vi "TTA_MATLAB_Set_MATLAB_Path.vi"(8 "error in":errorcluster, 11 "MATLAB Directory":path=path "C:/Users/Alex.Minicozzi.NJ01/Documents/LabVIEW Data/BDS_MATLAB/ViennaGUI") -> (0 "error out":errorcluster)   [LabVIEW 2016]
uses:
  TTA_Globals/Test_Environment.vi
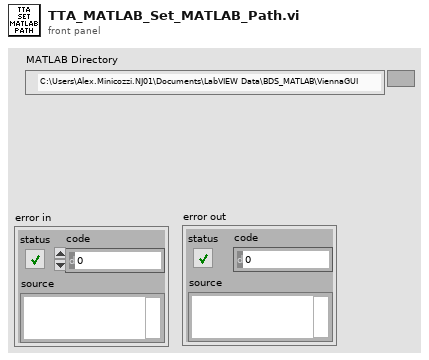
[diagram p1: front panel]
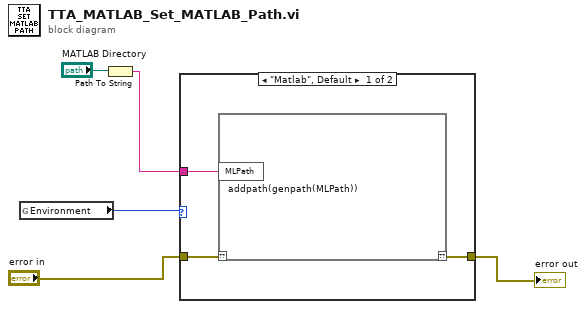
[diagram p0: block diagram]
diagram:
  n1 = global read "Test_Environment.vi" "Environment"() -> (w1:enum16{"Matlab", "LabVIEW"})
  n2 = Path To String(path="MATLAB Directory") -> (string=w2:string)
  n3 = case shown="\"Matlab\", Default" w1 {
    tunnel: "error in" -> [w8 w9]
    tunnel: [w7 w9] -> w4
    tunnel: w2 -> [w6 _]
    frame "Matlab", Default {
      n4 = script code="addpath(genpath(MLPath))"("??"=w8, "MLPath"=w6) -> ("??"=w7:errorcluster)
    }
    frame "LabVIEW" {
    }
  }
  "error out" <- w4
